vi "Archiver.Find.vi"(8 "error in":errorcluster, 9 "Check interval [min] (1)":dbl=1.0 format="%#_13g") -> (0 "error out":errorcluster, 2 "files to remove":path[](array[path]))   [LabVIEW 2016]
uses:
  tools/EventLog/EventLog.EventSource.ctl
  tools/Translator/Translator.Message.ctl
  tools/Config/Config.Global.vi
  Global/ApplicationGlobal.vi
  Drivers/Keyence/LowLevel/Keyence.Global.vi
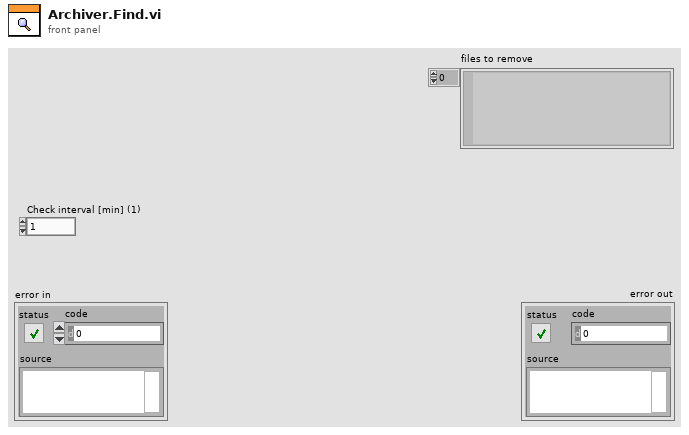
[diagram p1: front panel]
types:
  T1 = typedef "Translator.Message.ctl" = enum16{"-", "Event confirmed", "Log out", "Log in", "Shutdown", "Cancel", "Start", "Begin time", "End time", "Duration", "Service Mode", "Ignore Results", "Serial Format", "On", "Off", "OK", "NOK", "NOK %s", "Home", "Work", "Close", "Open", "In progress...", "Missing", "Empty", "Hardware failure", "Initial", "Default", "Total", "Out of range", "Free disk space is below 1GB - contact technician", "Error %d >> %s", "Error %d >> %s >> %s", "Msg %d >> %s", "Laser msg %d %s", "Laser cmd error %s %d", "Laser cmd failed %s", "Laser cmd warning %s", "Laser disconnected", "Laser status %s", "Laser already started", "Laser job unkonwn %s", "Laser job missing %s", "Laser job select failure %s", "Unable to start laser printing (%s)", "Unable to stop laser printing (%s)", "Laser marking aborted", "Laser marking timeout", "Unable to reset Laser Interlock (%s)", "Unable to trigger Laser. Laser not ready (%s)", "Laser job '%s' coordinates not configured", "Starting %s", "Quitting %s", "Configured", "Initializing", "Quitting", "Loading", "Loaded %d results", "Loaded %d events", "Running", "Stopped", "Summary", "Laser", "Do you want to continue?", "Do you want to delete the configuration?", "The configuration is being used by an order. Unable to delete!", "Press confirm button", "Station is not based. Do you want to exit?", "Station requires changeover. Do you want to run the test?", "Test options are not set as default. Do you want to continue?", "Formatting of WabcoNo is disabled. Do you want to continue?", "Product not detected. Do you want to continue?", "Product scan failed. Do you want to continue?", "Calibration", "Log out?", "System", "All", "IDLE", "Translating...%s", "Not found", "Alarm %s", "Run", "Skip", "Abort", "Repeat", "Please wait...", "Database disconnected", "Database disconnected - changeover disabled!", "Login to database successful", "Login to database failed: %d; %s", "Unable to check the product status of reference %d - database disconnected", "Unable to set the product status of reference %d - database disconnected", "Variant file backup %s", "Read variant (%s)", "Result", "Station armed!", "Station requires changeover!", "Select reference number...", "EMERGENCY BUTTON - press Control button", "EMERGENCY DOOR - press Control button", "Resetting Emergency...", "Unable to reset safety circuit - Emergency Button pressed", "Unable to reset safety circuit - Emergency Side Door open", "Station not based", "Station based", "Station not empty", "Station basing...", "No order", "Press Start to begin new order", "Scanning new order", "Order NOK. Correct or scan again", "Order OK. Press Accept", "Order ready", "Revolver incorrect", "Fork incorrect", "Revolver missing", "Revolver empty", "Container missing", "Offline results", "Offline statistics", "Updating statistics %.1f %%", "DMC Configurator", "Door open", "Close the front door", "Press start button", "Done. Open the front door", "Running...", "Running...%.1f %%", "Pause %s", "Pause %s. NOK container missing", "Pause %s. OK container missing", "Pause %s. Revolver empty", "Pause %s. Revolver missing", "Pause %s. Revolver incorrect", "Pause %s. Fork missing", "Pause %s. Fork incorrect", "Pause %s. Too many failures", "Pause %s. Unloading failure", "Pause %s. One slot is not working", "Pause %s. Part order is done. Empty OK container", "Pause %s. Unable to move product to slot", "Pause %s. Unable to move back product pusher", "Pause %s. Unable to lift product", "Pause %s. Unable to move back product lifter", "Pause %s. Unable to move product arm to Work", "Pause %s. Unable to move product arm to NOK", "Pause %s. Unable to move product arm to OK", "Pause %s. Unable to unsuck the NOK product", "Pause %s. Unable to drop the NOK product", "Pause %s. Product OK missing", "Pause %s. Unable to unsuck the OK product", "Pause %s. Unable to drop the OK product", "Stopping...", "File '%s' is missing", "File '%s' is broken", "File '%s' is running", "Log file started (%s)", "Log file ended (%s)", "Log file stopped (%s)", "Log file ignored (%s)", "Log file exported (%s)", "Log file export failed (%s)", "Wrong serial number in log file", "Wrong reference number in log file", "Test steps are missing", "%s = %.3f", "Process param '%s' not found in DB", "Process param '%s' wrong order", "Process param '%s' value %.3f out of limits (%.3f; %.3f)", "Step%d param '%s' not found in DB", "Step%d param '%s' wrong order", "Step%d param '%s' value %.3f out of limits (%.3f; %.3f)", "Step%d EV '%s' not found in DB", "Step%d EV '%s' wrong order", "\"%s\" not found in DB", "\"%s\" wrong order", "\"%s\" value %.3f out of limits (%.3f; %.3f)", "\"%s\" not found in software", "Process init (%s)", "Process started", "Process restarted", "Process run", "Process done", "Process done - remove OK container", "Process aborted", "Process aborted at work", "Process aborted at home", "Process error", "Process error at home", "Process error at work", "Process close", "Process pause", "Process continue", "Process door open", "Process door close", "Process pause at slot %s due to %s", "Select plate from the order to process", "Do you want to start the process?", "Do you want to continue the process?", "There is unfinished order. Do you want to put the new order?", "Product %s %d OK", "Product %s %d NOK", "Unable to unload the slot %s. Product missing in the slot", "Unable to unload the slot %s. Product already in the arm", "Unable to accept the product as OK. Product missing in slot %s", "Unable to accept the product as OK. Product could not drop into the container at slot %s", "Unable to accept the product as NOK. Product could not drop into the container at slot %s", "Scan failed. Error %s", "Scan failed. Scanner disconnected", "Scan failed. Wrong Wabco number %d, limit (%d,%d)", "Scan failed. Wrong serial number %d, limit (%d,%d)", "Scan failed. Wrong date %d, limit (%d,%d)", "Scan failed. Wrong product wabco number %d (expected %d)", "Scan failed. Wrong product serial number %d (expected > 0)", "Scan OK %s", "Scan failed. Unable to determine table position (%s)", "Scan failed. Timeout", "Tune failed. Scanner disconnected", "Tune failed. Timeout", "%s = %d", "%s = %d->%d", "Unable to set %s = %.2f - Air Pressure Inside off", "Unable to set digital output '%s' = %d", "Unable to activate air pressure inside - timeout", "Unable to activate air pressure inside - aborted", "Unable to switch on Air Main Valve - Air Pressure Inlet off", "Unable to switch on Air Main Valve - Door open", "Unable to switch off Air Main Valve - timeout", "Unable to switch off Air Main Valve - aborted", "Unable to rotate Table - timeout", "Unable to rotate Table - aborted", "Unable to rotate Table - Product Move not in Home position", "Unable to rotate Table - Air Pressure Inside off", "Unable to rotate Table - Product Lift A not in Home position", "Unable to rotate Table - Product Lift B not in Home position", "Unable to rotate Table - unlock before movement timeout", "Unable to rotate Table - lock after movement timeout", "Unable to move Table Lock to %s position - timeout", "Unable to move Table Lock to %s position - aborted", "Unable to move Table Lock to %s position - Air Pressure Inside off", "Unable to move Table Lock to %s position - Table not in position", "Unable to move Product Lift A to %s position - timeout", "Unable to move Product Lift B to %s position - timeout", "Unable to move Product Lift A to %s position - aborted", "Unable to move Product Lift B to %s position - aborted", "Unable to move Product Lift A to %s position - Air Pressure Inside off", "Unable to move Product Lift B to %s position - Air Pressure Inside off", "Unable to move Product Lift A to %s position - Table not locked", "Unable to move Product Lift B to %s position - Table not locked", "Unable to move Product Lift A to %s position - Product Arm not in Work position", "Unable to move Product Lift B to %s position - Product Arm not in Work position", "Unable to set Product Suction Gripper %s to %s - timeout", "Unable to set Product Suction Gripper %s to %s - aborted", "Unable to set Product Suction Gripper %s to %s - Air Pressure Inside off", "Unable to set Product Suction Gripper %s to %s - Table slot unkown", "Unable to move Product Arm to %s position - timeout", "Unable to move Product Arm to %s position - aborted", "Unable to move Product Arm to %s position - Air Pressure Inside off", "Unable to move Product Arm to %s position - Product Lift A not in Home position", "Unable to move Product Arm to %s position - Product Lift B not in Home position", "Unable to move Product to %s position - timeout", "Unable to move Product to %s position - aborted", "Unable to move Product to %s position - Air Pressure Inside off", "Unable to move Product to %s position - Table not in position"}
  T2 = typedef "EventLog.EventSource.ctl" = enum16{"All", "Gui", "Ref", "File", "Arch", "Seq", "CPX", "DB", "Laser", "Scan.P", "Scan.O"}
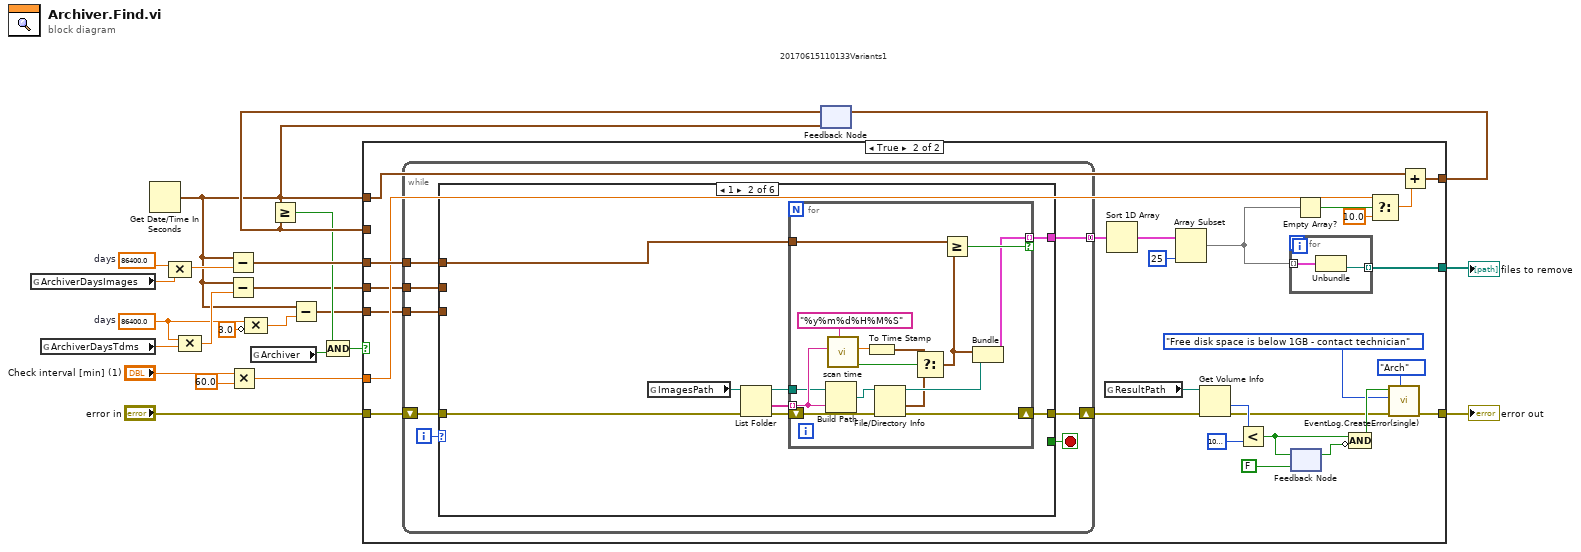
[diagram p0: block diagram]
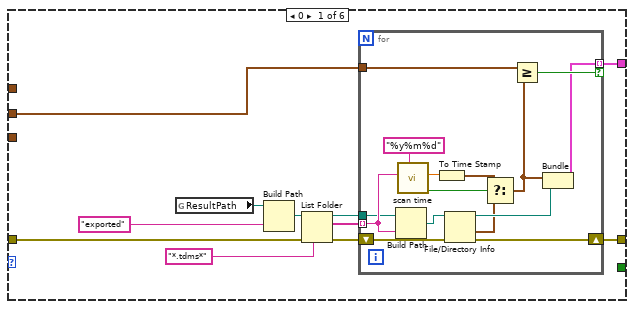
[diagram p3: hidden frame]
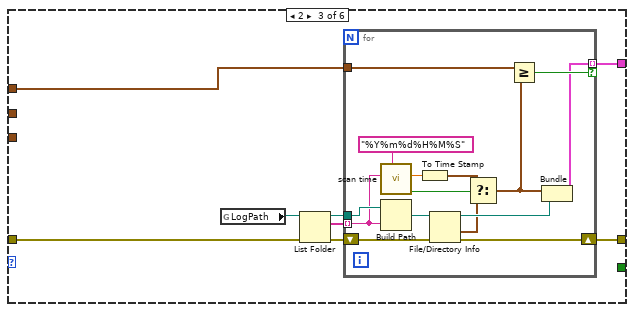
[diagram p4: hidden frame]
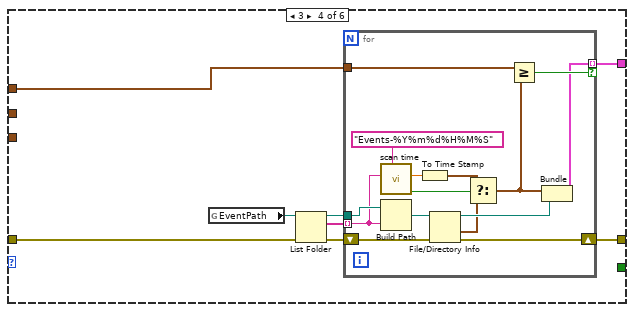
[diagram p5: hidden frame]
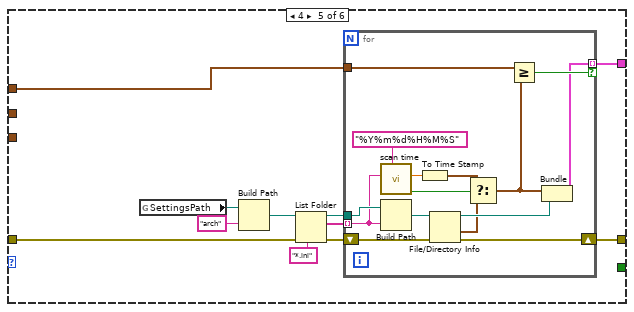
[diagram p6: hidden frame]
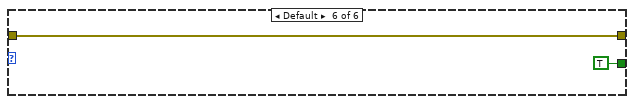
[diagram p7: hidden frame]
diagram:
  w3 = 86400.0  # days
  w19 = 86400.0  # days
  # "20170615110133Variants1"
  n1 = global read "Config.Global.vi" "ArchiverDaysImages"() -> (w6:dbl)
  n2 = global read "Config.Global.vi" "ArchiverDaysTdms"() -> (w7:dbl)
  n3 = Get Date/Time In Seconds() -> (seconds since 1Jan1904=w5:timestamp)
  n4 = Compound Arithmetic op=MULTIPLY(w19, w6) -> (w18:dbl)
  n5 = Compound Arithmetic op=MULTIPLY(w3, w7) -> (w10:dbl)
  n6 = Subtract(x=w5, y=w18) -> (x-y=w17:timestamp)
  n7 = Subtract(x=w5, y=w10) -> (x-y=w9:timestamp)
  n8 = Multiply(x="Check interval [min] (1)", y=60.0 ("x")) -> (x*y=w14:dbl)
  n9 = Compound Arithmetic op=MULTIPLY(w3, invert 3.0 ("value")) -> (w1:dbl)
  n10 = global read "Config.Global.vi" "Archiver"() -> (w11:bool)
  n11 = Subtract(x=w5, y=w1) -> (x-y=w4:timestamp)
  n12 = feedback #1(w5) -> (w21:timestamp)
  n13 = Greater Or Equal?(x=w5, y=w21) -> (x >= y?=w12:bool)
  n14 = Compound Arithmetic op=AND(w12, w11) -> (w13:bool)
  n15 = case shown="True" w13 {
    tunnel: "error in" -> [w24 w52]
    tunnel: w5 -> [_ w26]
    tunnel: [w25 w48] -> w22
    tunnel: w21 -> [w25 _]
    tunnel: [w24 w30] -> w20
    tunnel: w17 -> [_ w51]
    tunnel: w14 -> [_ w50]
    tunnel: [_ w42] -> w8
    tunnel: w9 -> [_ w45]
    tunnel: w4 -> [_ w27]
    frame False {
    }
    frame True {
      n16 = while {
        tunnel: [w61] -> w46 mode=concatenating
        tunnel: w51 -> [w59]
        shift-right: [w60] -> w39
        shift-left: w52 -> [w62]
        tunnel: w45 -> [w56]
        tunnel: w27 -> [w55]
        i -> [w58]
        stop <- w57 stop-if-true
        n17 = case shown="1" w58 {
          tunnel: w62 -> [w73 w96 w116 w139 w165 w184]
          tunnel: [w70 w94 w114 w137 w163 _] -> w61
          tunnel: [w68 w93 w115 w138 w164 w184] -> w60
          tunnel: w59 -> [_ w91 w113 w136 w162 _]
          tunnel: [_ _ _ _ _ TRUE] -> w57
          tunnel: w56 -> [w66 _ _ _ _ _]
          tunnel: w55 -> [_ _ _ _ _ _]
          frame 0 {
            n18 = global read "ApplicationGlobal.vi" "ResultPath"() -> (w64:path)
            n19 = Build Path(base path=w64, name or relative path="exported") -> (appended path=w63:path)
            n20 = List Folder(path=w63, pattern="*.tdms*", error in=w73) -> (path out=w67:path, filenames=w72:string[], error out=w71:errorcluster)  [unwired: 1 in, 1 out]
            n21 = for {
              tunnel: w72 -> [w81] mode=indexing
              tunnel: w67 -> [w80]
              shift-right: [w87] -> w68
              shift-left: w71 -> [w88]
              tunnel: w66 -> [w86]
              tunnel: [w83] -> w70 mode=indexing if=w85
              n22 = Build Path(base path=w80, name or relative path=w81) -> (appended path=w84:path)
              n23 = call "scan time.vi"("time format string"="%y%m%d", "formatted time string"=w81) -> ("ok?"=w77:bool, "lv time (UTC)"=w78:dbl)  [unwired: 5 in, 3 out]
              n24 = To Time Stamp(1:w78) -> (0:w76:timestamp)
              n25 = File/Directory Info(path=w84, error in=w88) -> (path out=w82:path, last mod=w75:timestamp, error out=w87:errorcluster)  [unwired: 4 out]
              n26 = Select(t=w76, s=w77, f=w75) -> (s? t:f=w74:timestamp)
              n27 = Greater Or Equal?(x=w86, y=w74) -> (x >= y?=w85:bool)
              n28 = Bundle("last mod"=w74, "path out"=w82) -> (w83:cluster{"last mod":timestamp, "path out":path})  [unwired: 1 in]
            }
          }
          frame 1 {
            n29 = global read "ApplicationGlobal.vi" "ImagesPath"() -> (w90:path)
            n30 = List Folder(path=w90, error in=w96) -> (path out=w92:path, folder names=w89:string[], error out=w95:errorcluster)  [unwired: 2 in, 1 out]
            n31 = for {
              tunnel: w89 -> [w104] mode=indexing
              tunnel: w92 -> [w103]
              shift-right: [w110] -> w93
              shift-left: w95 -> [w111]
              tunnel: w91 -> [w109]
              tunnel: [w106] -> w94 mode=indexing if=w108
              n32 = Build Path(base path=w103, name or relative path=w104) -> (appended path=w107:path)
              n33 = call "scan time.vi"("time format string"="%y%m%d%H%M%S", "formatted time string"=w104) -> ("ok?"=w100:bool, "lv time (UTC)"=w101:dbl)  [unwired: 5 in, 3 out]
              n34 = To Time Stamp(1:w101) -> (0:w99:timestamp)
              n35 = File/Directory Info(path=w107, error in=w111) -> (path out=w105:path, last mod=w98:timestamp, error out=w110:errorcluster)  [unwired: 4 out]
              n36 = Select(t=w99, s=w100, f=w98) -> (s? t:f=w97:timestamp)
              n37 = Greater Or Equal?(x=w109, y=w97) -> (x >= y?=w108:bool)
              n38 = Bundle("last mod"=w97, "path out"=w105) -> (w106:cluster{"last mod":timestamp, "path out":path})  [unwired: 1 in]
            }
          }
          frame 2 {
            n39 = global read "Keyence.Global.vi" "LogPath"() -> (w112:path)
            n40 = List Folder(path=w112, error in=w116) -> (path out=w118:path, filenames=w117:string[], error out=w119:errorcluster)  [unwired: 2 in, 1 out]
            n41 = for {
              tunnel: w117 -> [w124] mode=indexing
              tunnel: w118 -> [w131]
              shift-right: [w133] -> w115
              shift-left: w119 -> [w134]
              tunnel: w113 -> [w132]
              tunnel: [w128] -> w114 mode=indexing if=w130
              n42 = call "scan time.vi"("time format string"="%Y%m%d%H%M%S", "formatted time string"=w124) -> ("ok?"=w123:bool, "lv time (UTC)"=w126:dbl)  [unwired: 5 in, 3 out]
              n43 = Build Path(base path=w131, name or relative path=w124) -> (appended path=w129:path)
              n44 = To Time Stamp(1:w126) -> (0:w125:timestamp)
              n45 = File/Directory Info(path=w129, error in=w134) -> (path out=w127:path, last mod=w122:timestamp, error out=w133:errorcluster)  [unwired: 4 out]
              n46 = Select(t=w125, s=w123, f=w122) -> (s? t:f=w121:timestamp)
              n47 = Greater Or Equal?(x=w132, y=w121) -> (x >= y?=w130:bool)
              n48 = Bundle("last mod"=w121, "path out"=w127) -> (w128:cluster{"last mod":timestamp, "path out":path})  [unwired: 1 in]
            }
          }
          frame 3 {
            n49 = global read "ApplicationGlobal.vi" "EventPath"() -> (w135:path)
            n50 = List Folder(path=w135, error in=w139) -> (path out=w141:path, filenames=w140:string[], error out=w142:errorcluster)  [unwired: 2 in, 1 out]
            n51 = for {
              tunnel: w140 -> [w147] mode=indexing
              tunnel: w141 -> [w154]
              shift-right: [w156] -> w138
              shift-left: w142 -> [w157]
              tunnel: w136 -> [w155]
              tunnel: [w151] -> w137 mode=indexing if=w153
              n52 = call "scan time.vi"("time format string"="Events-%Y%m%d%H%M%S", "formatted time string"=w147) -> ("ok?"=w146:bool, "lv time (UTC)"=w149:dbl)  [unwired: 5 in, 3 out]
              n53 = Build Path(base path=w154, name or relative path=w147) -> (appended path=w152:path)
              n54 = To Time Stamp(1:w149) -> (0:w148:timestamp)
              n55 = File/Directory Info(path=w152, error in=w157) -> (path out=w150:path, last mod=w145:timestamp, error out=w156:errorcluster)  [unwired: 4 out]
              n56 = Select(t=w148, s=w146, f=w145) -> (s? t:f=w144:timestamp)
              n57 = Greater Or Equal?(x=w155, y=w144) -> (x >= y?=w153:bool)
              n58 = Bundle("last mod"=w144, "path out"=w150) -> (w151:cluster{"last mod":timestamp, "path out":path})  [unwired: 1 in]
            }
          }
          frame 4 {
            n59 = global read "ApplicationGlobal.vi" "SettingsPath"() -> (w160:path)
            n60 = Build Path(base path=w160, name or relative path="arch") -> (appended path=w159:path)
            n61 = List Folder(path=w159, pattern="*.ini", error in=w165) -> (path out=w167:path, filenames=w166:string[], error out=w168:errorcluster)  [unwired: 1 in, 1 out]
            n62 = for {
              tunnel: w166 -> [w173] mode=indexing
              tunnel: w167 -> [w180]
              shift-right: [w182] -> w164
              shift-left: w168 -> [w183]
              tunnel: w162 -> [w181]
              tunnel: [w177] -> w163 mode=indexing if=w179
              n63 = call "scan time.vi"("time format string"="%Y%m%d%H%M%S", "formatted time string"=w173) -> ("ok?"=w172:bool, "lv time (UTC)"=w175:dbl)  [unwired: 5 in, 3 out]
              n64 = Build Path(base path=w180, name or relative path=w173) -> (appended path=w178:path)
              n65 = To Time Stamp(1:w175) -> (0:w174:timestamp)
              n66 = File/Directory Info(path=w178, error in=w183) -> (path out=w176:path, last mod=w171:timestamp, error out=w182:errorcluster)  [unwired: 4 out]
              n67 = Select(t=w174, s=w172, f=w171) -> (s? t:f=w170:timestamp)
              n68 = Greater Or Equal?(x=w181, y=w170) -> (x >= y?=w179:bool)
              n69 = Bundle("last mod"=w170, "path out"=w176) -> (w177:cluster{"last mod":timestamp, "path out":path})  [unwired: 1 in]
            }
          }
          frame Default {
          }
        }
      }
      n70 = global read "ApplicationGlobal.vi" "ResultPath"() -> (w38:path)
      n71 = Sort 1D Array(array=w46) -> (sorted array=w44:cluster{"last mod":timestamp, "path out":path}[])
      n72 = Array Subset(array=w44, length=25) -> (w41:cluster{"last mod":timestamp, "path out":path}[])  [unwired: 1 in]
      n73 = Get Volume Info(8:w39, 11:w38) -> (0:w31:errorcluster, 1:w37:i64)  [unwired: 4 out]
      n74 = Less?(x=w37, y=i64 1000000000) -> (x < y?=w35:bool)
      n75 = for {
        tunnel: w41 -> [w54] mode=indexing
        tunnel: [w53] -> w42 mode=indexing
        n76 = Unbundle(w54) -> ("path out"=w53:path)  [unwired: 1 out]
      }
      n77 = feedback-in #2(w35) -> ()
      n78 = feedback #2(FALSE) -> (w33:bool)
      n79 = Empty Array?(array=w41) -> (empty?=w40:bool)
      n80 = Compound Arithmetic op=AND(w35, invert w33) -> (w32:bool)
      n81 = Select(t=w50, s=w40, f=10.0) -> (s? t:f=w49:dbl)
      n82 = call "EventLog.CreateError(single).vi"("Source (All)"=EventLog.EventSource."Arch", "error in"=w31, "msg"=Translator.Message."Free disk space is below 1GB - contact technician", "create (T)"=w32) -> ("error out"=w30:errorcluster)  [unwired: 7 in]
      n83 = Add(x=w26, y=w49) -> (x+y=w48:timestamp)
    }
  }
  "error out" <- w20
  "files to remove" <- w8
  n84 = feedback-in #1(w22) -> ()
